vi "UnscentedKalmanFilter_New_FuncGroup.vi"(0 "addFuncXExtra":variant, 3 "MeanFuncX":T2, 4 "AddFuncX":T2, 5 "MeanFuncXExtra":variant, 6 "residualFuncYExtra":variant, 7 "MeanFuncY":T2, 8 "ResidualFuncY":T2, 9 "residualFuncXExtra":variant, 10 "ResidualFuncX":T2, 11 "MeanFuncYExtra":variant) -> (1 "Error":bool, 2 "UNSCENTED_KALMAN_NEW_FUNC_GROUP":T1)   [LabVIEW 2019, in "Trajectory_Library.lvlib"]
doc: "Creates a new LINEAR SYSTEM data cluster with the specified values. \n\n\nInputs: \n - XXX -- XXX.\n\nOutputs:\n - XXX -- XXX."
uses:
  Trajectory_Library.lvlib
  BiFun_Matrix_FUNC_TYPE.ctl
  UNSCENTED_KALMAN_NEW_FUNC_GROUP.ctl
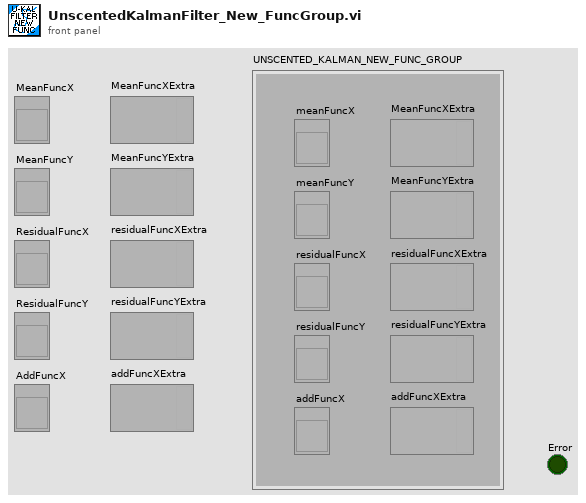
[diagram p1: front panel]
types:
  T1 = typedef "Trajectory_Library.lvlib/UNSCENTED_KALMAN_NEW_FUNC_GROUP.ctl" = cluster{"meanFuncX":T2, "meanFuncY":T2, "residualFuncX":T2, "residualFuncY":T2, "addFuncX":T2, "MeanFuncXExtra":variant, "MeanFuncYExtra":variant, "residualFuncXExtra":variant, "residualFuncYExtra":variant, "addFuncXExtra":variant}
  T2 = typedef "Trajectory_Library.lvlib/BiFun_Matrix_FUNC_TYPE.ctl" = refnum<vi>
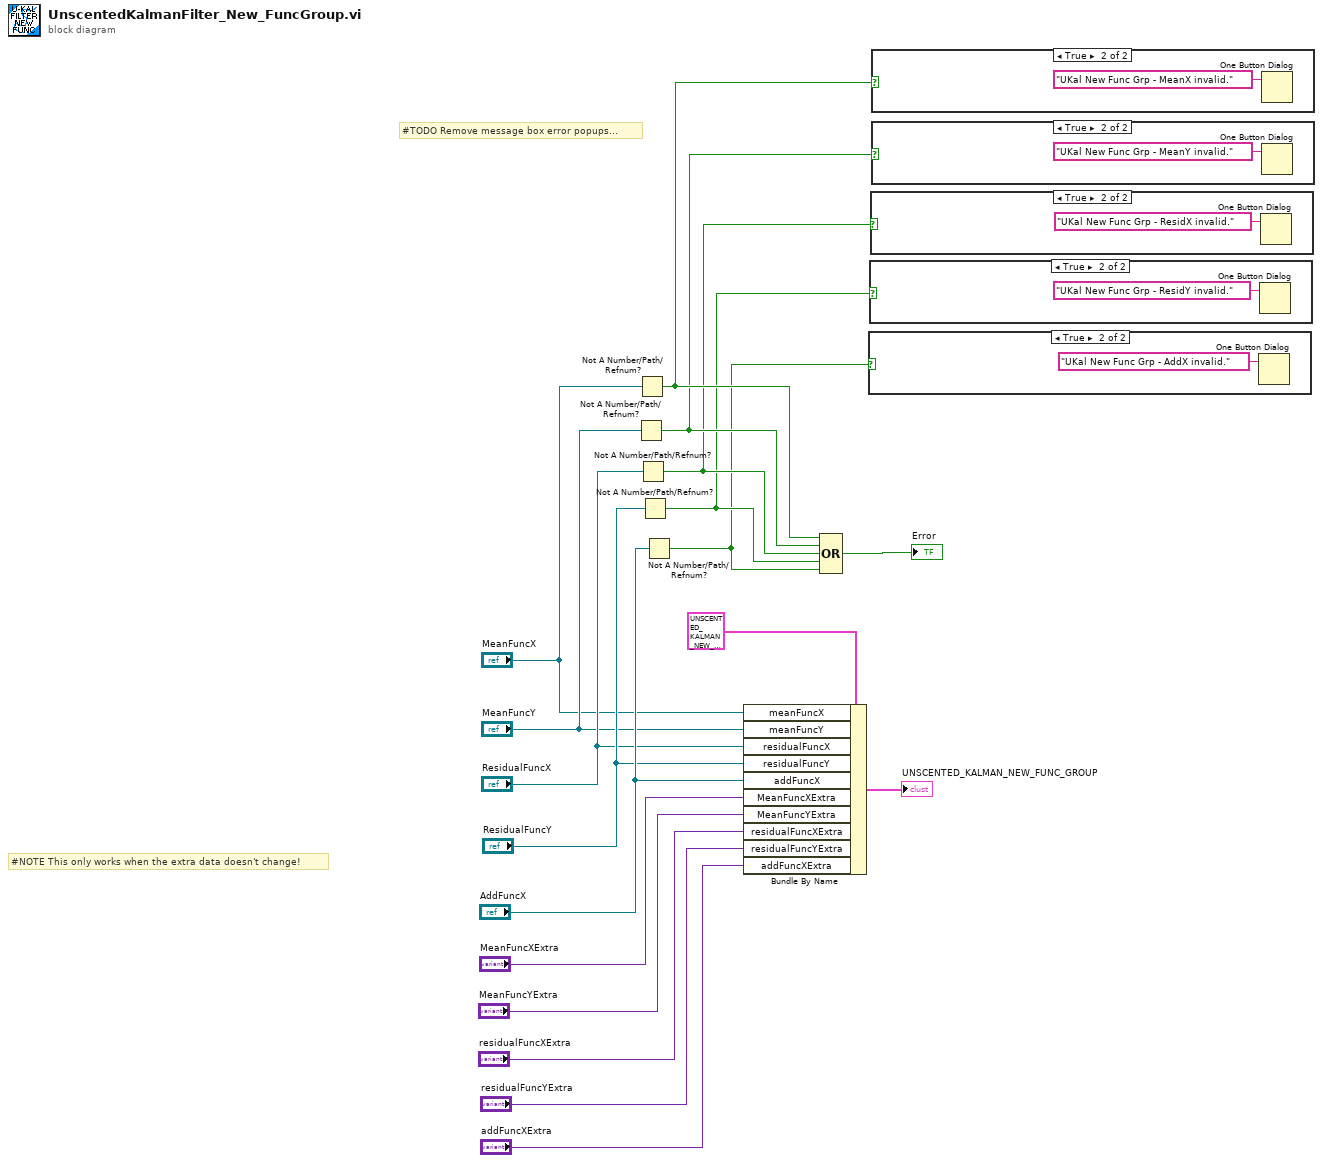
[diagram p0: block diagram]
diagram:
  # "#TODO Remove message box error popups..."
  # "#NOTE This only works when the extra data doesn't change!"
  n1 = Not A Number/Path/Refnum?(number/path/refnum="MeanFuncY") -> (NaN/Path/Refnum?=w4:bool)
  n2 = Not A Number/Path/Refnum?(number/path/refnum="MeanFuncX") -> (NaN/Path/Refnum?=w5:bool)
  n3 = Not A Number/Path/Refnum?(number/path/refnum="ResidualFuncX") -> (NaN/Path/Refnum?=w3:bool)
  n4 = Not A Number/Path/Refnum?(number/path/refnum="ResidualFuncY") -> (NaN/Path/Refnum?=w2:bool)
  n5 = Not A Number/Path/Refnum?(number/path/refnum="AddFuncX") -> (NaN/Path/Refnum?=w1:bool)
  n6 = Bundle By Name(cluster=T1 {"meanFuncX"=refnum, "meanFuncY"=refnum, "residualFuncX"=refnum, "residualFuncY"=refnum, "addFuncX"=refnum, "MeanFuncXExtra"=variant, "MeanFuncYExtra"=variant, "residualFuncXExtra"=variant, "residualFuncYExtra"=variant, "addFuncXExtra"=variant} ("UNSCENTED_KALMAN_FILTER_FUNC_GROUP"), "meanFuncX"="MeanFuncX", "meanFuncY"="MeanFuncY", "residualFuncX"="ResidualFuncX", "residualFuncY"="ResidualFuncY", "addFuncX"="AddFuncX", "MeanFuncXExtra"="MeanFuncXExtra", "MeanFuncYExtra"="MeanFuncYExtra", "residualFuncXExtra"="residualFuncXExtra", "residualFuncYExtra"="residualFuncYExtra", "addFuncXExtra"="addFuncXExtra") -> (→"UNSCENTED_KALMAN_NEW_FUNC_GROUP":T1)
  n7 = Compound Arithmetic op=OR(w5, w4, w3, w2, w1) -> (→"Error":bool)
  n8 = case shown="True" w1 {
    frame False {
    }
    frame True {
      n9 = One Button Dialog(message="UKal New Func Grp - AddX invalid.") -> ()  [unwired: 1 in, 1 out]
    }
  }
  n10 = case shown="True" w2 {
    frame False {
    }
    frame True {
      n11 = One Button Dialog(message="UKal New Func Grp - ResidY invalid.") -> ()  [unwired: 1 in, 1 out]
    }
  }
  n12 = case shown="True" w3 {
    frame False {
    }
    frame True {
      n13 = One Button Dialog(message="UKal New Func Grp - ResidX invalid.") -> ()  [unwired: 1 in, 1 out]
    }
  }
  n14 = case shown="True" w5 {
    frame False {
    }
    frame True {
      n15 = One Button Dialog(message="UKal New Func Grp - MeanX invalid.") -> ()  [unwired: 1 in, 1 out]
    }
  }
  n16 = case shown="True" w4 {
    frame False {
    }
    frame True {
      n17 = One Button Dialog(message="UKal New Func Grp - MeanY invalid.") -> ()  [unwired: 1 in, 1 out]
    }
  }
